vi "Actor Core.vi"(8 "error in":errorcluster, 11 "Controller in":refnum<class "Controller.lvclass">) -> (0 "error out":errorcluster, 3 "Actor out":refnum<class "Actor.lvclass">)   [LabVIEW 2022 SP3, in "Controller.lvlib" / "Controller.lvclass"]
doc: "(<B>Filename</B>: Actor Framework.lvlib:Actor.lvclass:Actor Core.vi)\n\nReceives messages to the actor, reacts to them, and initiates any error handling that may shut the actor down.\n\nDescendant classes may override this VI to append parallel tasks for the actor to complete while it handles messages. Overrides use the Call Parent Class Method node."
uses:
  Controller.lvclass
  C:/Program Files (x86)/National Instruments/LabVIEW 2022/vi.lib/ActorFramework/Actor/Actor.lvclass
  <vilib>/ActorFramework/Actor/Actor.lvclass
  Cli/Cli/Cli.lvclass
  Controller.lvclass/Controller.ctl
  <vilib>/ActorFramework/Message Enqueuer/Message Enqueuer.lvclass
  LoggingActor/Source/LoggingActor/LoggingActor/LoggingActor.lvclass
  Gui/Gui/Gui.lvclass
  Gui/Gui Messages/ShowFrontPanel Msg/ShowFrontPanel Msg.lvclass
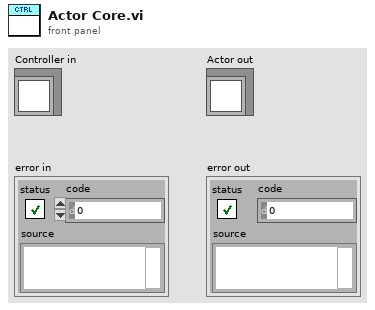
[diagram p1: front panel]
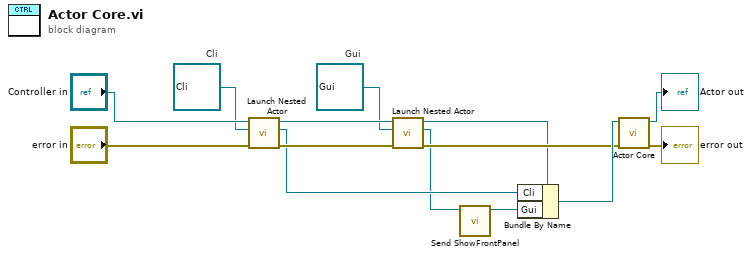
[diagram p0: block diagram]
diagram:
  w2 = refnum<class "Gui.lvclass"> refnum  # Gui
  w9 = refnum<class "Cli.lvclass"> refnum  # Cli
  n1 = call <vilib>:"Launch Nested Actor.vi"("error in (no error)"="error in", "Nested Actor"=w9, "Caller Actor in"="Controller in") -> ("error out"=w11:errorcluster, "Nested Actor's Enqueuer"=w8:refnum<class "Message Enqueuer.lvclass">, "Caller Actor out"=w5:refnum<class "Controller.lvclass">)  [unwired: 6 in]
  n2 = call <vilib>:"Launch Nested Actor.vi"("error in (no error)"=w11, "Nested Actor"=w2, "Caller Actor in"=w5) -> ("error out"=w6:errorcluster, "Nested Actor's Enqueuer"=w1:refnum<class "Message Enqueuer.lvclass">, "Caller Actor out"=w4:refnum<class "Controller.lvclass">)  [unwired: 6 in]
  n3 = call "Send ShowFrontPanel.vi"("Message Enqueuer"=w1) -> ("Message Enqueuer out"=w3:refnum<class "Message Enqueuer.lvclass">)  [unwired: 9 in, 1 out]
  n4 = Bundle By Name(cluster=w4, "Cli"=w8, "Gui"=w3) -> (w7:refnum<class "Controller.lvclass">)
  n5 = call-parent "Actor Core.vi"("error in"=w6, "Actor in"=w7) -> ("error out"=→"error out":errorcluster, "Actor out"=→"Actor out":refnum<class "Actor.lvclass">)  [unwired: 8 in]
